vi "Cleanup.vi"(8 "error in (no error)":errorcluster, 11 "VISA Client in":refnum<class "Serial Client.lvclass">) -> (0 "error out":errorcluster)   [LabVIEW 2020, in "Stream-Serial.lvlib" / "Serial Client.lvclass"]
doc: "Closes the connection if it's open and cleans up resources used by the class. This should always be called for any created instances when they're no longer needed to prevent reference leaks and memory usage accumulation in long running applications."
uses:
  Serial Client.lvclass
  Serial Client.lvclass/Serial Client.ctl
  <vilib>/IlluminatedG/lv-stream/Connection/Connection.lvclass
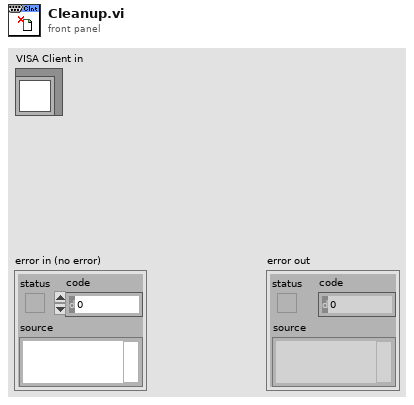
[diagram p1: front panel]
types:
  T1 = typedef "Stream-Serial.lvlib/Command Queue.ctl" = refnum<queue>
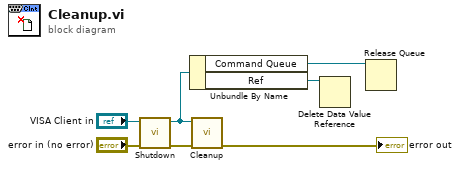
[diagram p0: block diagram]
diagram:
  n1 = call "Shutdown.vi"("error in (no error)"="error in (no error)", "VISA Client in"="VISA Client in") -> ("error out"=w5:errorcluster, "VISA Client out"=w4:refnum<class "Serial Client.lvclass">)  [unwired: 8 in]
  n2 = Unbundle By Name(w4) -> ("Command Queue"=w2:T1, "Ref"=w3:refnum<data-value>)
  n3 = call-parent "Cleanup.vi"("error in (no error)"=w5, "Connection in"=w4) -> ("error out"=→"error out":errorcluster)  [unwired: 9 in]
  n4 = Delete Data Value Reference(data value reference=w3) -> ()  [unwired: 1 in, 2 out]
  n5 = Release Queue(queue=w2) -> ()  [unwired: 2 in, 3 out]
